vi "Update Configuration.vi"(8 "error in (no error)":errorcluster, 10 "Parameters":T3, 11 "connection info":T4) -> (0 "error out":errorcluster, 1 "Timed Out?":bool, 2 "GetSettings":T1, 3 "connection info":T4)   [LabVIEW 2019, in "PID Control Host API.lvlib"]
uses:
  PID Control Host API.lvlib
  <vilib>/NI/STM/TCP/TCP Connection Info.ctl
  <vilib>/NI/STM/SubVIs/MetaDataElement.ctl
  Shared/Types/Update Parameters Message.ctl
  Shared/Types/Get Settings Message.ctl
  Shared/Types/Gain Schedule.ctl
  Shared/Control Addon Shared.lvlib
  <vilib>/NI/NIVS Addon Network Comm/Shared/NI VeriStand Addon Network Comm Shared.lvlib
  <vilib>/NI/STM/NI STM.lvlib
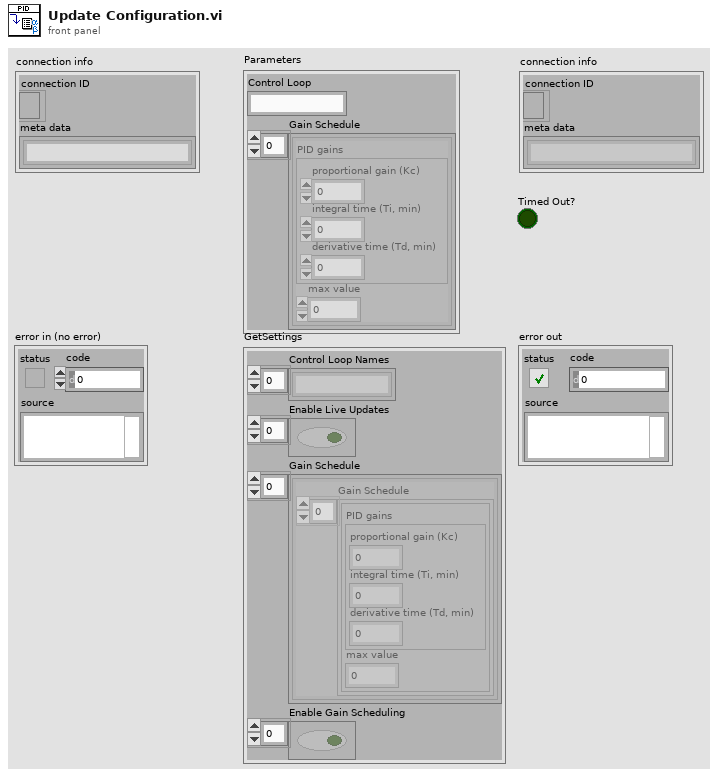
[diagram p1: front panel]
types:
  T1 = typedef "Control Addon Shared.lvlib/Get Settings Message.ctl" = cluster{"Control Loop Names":string[], "Enable Live Updates":bool[], "Gain Schedule":T2[], "Enable Gain Scheduling":bool[]}
  T2 = typedef "Control Addon Shared.lvlib/Gain Schedule.ctl" = cluster{"Gain Schedule":cluster{"PID gains":cluster{"proportional gain (Kc)":dbl, "integral time (Ti, min)":dbl, "derivative time (Td, min)":dbl}, "max value":dbl}[]}
  T3 = typedef "Control Addon Shared.lvlib/Update Parameters Message.ctl" = cluster{"Control Loop":string, "Gain Schedule":cluster{"PID gains":cluster{"proportional gain (Kc)":dbl, "integral time (Ti, min)":dbl, "derivative time (Td, min)":dbl}, "max value":dbl}[]}
  T4 = typedef "NI STM.lvlib/TCP Connection Info.ctl" = cluster{"connection ID":refnum<k5>, "meta data":T5[]}
  T5 = typedef "NI STM.lvlib/MetaDataElement.ctl" = string
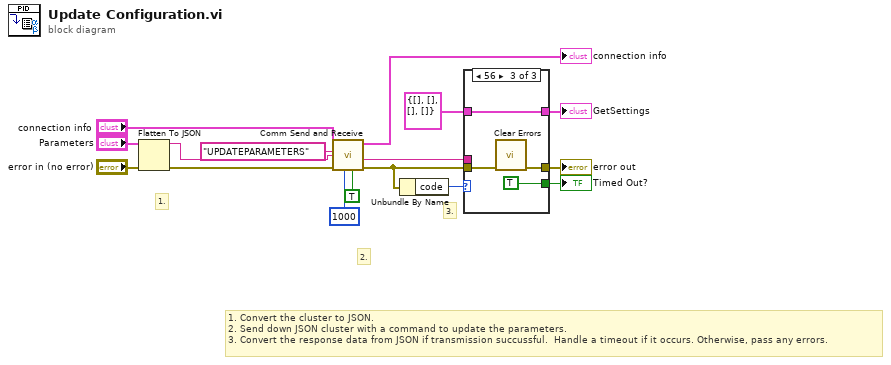
[diagram p0: block diagram]
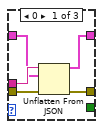
[diagram p2: hidden frame]
diagram:
  # "1. Convert the cluster to JSON.\n2. Send down JSON cluster with a command to update the parameters.\n3. Convert the response data from JSON if transmission succussful.  Handle a timeout if it occurs. Otherwise, pass any errors."
  # "3."
  # "2."
  # "1."
  n1 = Flatten To JSON(anything="Parameters", error in (no error)="error in (no error)") -> (JSON string=w6:string, 11:w5:errorcluster)  [unwired: 1 in]
  n2 = call <vilib>:"Comm Send and Receive.vi"("Resp Required?"=TRUE, "Timeout (ms)"=u32 1000 ("Timeout ms (5000)"), "error in (no error)"=w5, "Data"=w6, "Name"="UPDATEPARAMETERS", "connection info"="connection info") -> ("error out"=w4:errorcluster, "Data"=w2:string, "connection info"=→"connection info":T4)  [unwired: 2 in, 1 out]
  n3 = Unbundle By Name(w4) -> ("code"=w11:i32)
  n4 = case shown="56" w11 {
    tunnel: w2 -> [w21 _ _]
    tunnel: w4 -> [w20 w23 w24]
    tunnel: [w19 w23 w25] -> w13
    tunnel: [w18 w22 w27] -> w12
    tunnel: T1 {"Control Loop Names"=[], "Enable Live Updates"=[], "Gain Schedule"=[], "Enable Gain Scheduling"=[]} ("GetSettings") -> [w17 w22 w27]
    tunnel: [_ _ TRUE] -> w10
    frame 0 {
      n5 = Unflatten From JSON(JSON string=w21, type and defaults=w17, error in (no error)=w20) -> (value=w18:T1, error out=w19:errorcluster)  [unwired: 4 in]
    }
    frame Default {
    }
    frame 56 {
      n6 = call <vilib>:"Clear Errors.vi"("error in (no error)"=w24) -> ("error out"=w25:errorcluster)  [unwired: 5 in, 1 out]
    }
  }
  "error out" <- w13
  "Timed Out?" <- w10
  "GetSettings" <- w12
